vi "Elevator Controller.vi"(8 "error in":errorcluster) -> ()   [LabVIEW 2018]
doc: "This VI executes continuously carrying out the current operation and responding to updates or new operations. It will often contain the timing or control code that is difficult to place directly in TeleOp. This VI generally opens all sensors and motors and isolates the rest of the robot code from knowing how the operations are carried out."
uses:
  <vilib>/Rock Robotics/WPI/Framework/Completion Status.ctl
  Elevator Setpoints.ctl
  Elevator Operations.ctl
  <vilib>/Rock Robotics/WPI/ThirdParty/Phoenix-LabVIEW/Motor Controller/Controls/CTRE_Phoenix_MotorControl_FeedbackDevice.ctl
  <vilib>/Rock Robotics/WPI/ThirdParty/Phoenix-LabVIEW/Motor Controller/Controls/CTRE_Phoenix_MotorControl_LimitSwitchNormal.ctl
  <vilib>/Rock Robotics/WPI/ThirdParty/Phoenix-LabVIEW/Motor Controller/Controls/CTRE_Phoenix_MotorControl_LimitSwitchSource_Local.ctl
  <vilib>/Rock Robotics/WPI/ThirdParty/Phoenix-LabVIEW/Motor Controller/Controls/CTRE_Phoenix_MotorControl_ControlMode.ctl
  <vilib>/Rock Robotics/WPI/ThirdParty/Phoenix-LabVIEW/Motor Controller/Get/CTRE_Phoenix_MotorController_GetSelectedSensorData.vi
  <vilib>/Rock Robotics/Network Tables/NT Write Number.vi
  Elevator Published Globals.vi
  Framework/Robot Global Data.vi
  <vilib>/Rock Robotics/WPI/ThirdParty/Phoenix-LabVIEW/Motor Controller/Get/CTRE_Phoenix_MotorController_GetLimitSwitchStates.vi
  <vilib>/Rock Robotics/Network Tables/NT Write Boolean.vi
  <vilib>/Rock Robotics/WPI/ThirdParty/Phoenix-LabVIEW/Motor Controller/Get/CTRE_Phoenix_MotorController_GetClosedLoopData.vi
panel:
  in  "Time LimitDebounce":u32=500
  in  "ElevatorStopRange":dbl=20.0 format="%#_13g"
  out "Waveform Chart":i32(graph)
  out "inches":dbl=8.0
  out "% error":i32(graph)
  out "Position (Raw Sensor Units)":i32=208
  out "Waveform Chart 2":T1(graph)
  in  "Acceleration":i32=75
  in  "Cruise Velocity":i32=70
  in  "F":dbl=10.0
  in  "P":dbl=13.0
  in  "I":dbl
  in  "D":dbl
  in  "Interactive Values":T2={"Operation"=enum."LiftForTime", "Setpoint"=0.5, "Duration"=1.0, "Button"=FALSE}
  out "Current\nCmd":string="Started at  12:26:25.181\nDefault: Reserve,  S 0.0, D 0.000000"
  in  "Buttons":cluster{"Execute Cmd":bool, "Abort Cmd":bool}
  out "Command Timing":cluster{"Start Time (ms)":u32, "Iterations":i32}={"Start Time (ms)"=346916, "Iterations"=0}
  out "Status":T4=enum."Incomplete"
  # "Tip: It may be helpful to observe inputs and sensor values.\nYou may also want to display tuning or debugging controls."
  # "Interactive Command: You may fill in the settings for a command\nand schedule it with the Execute button. You can observe and abort\nany command while fine tuning the code for the controller."
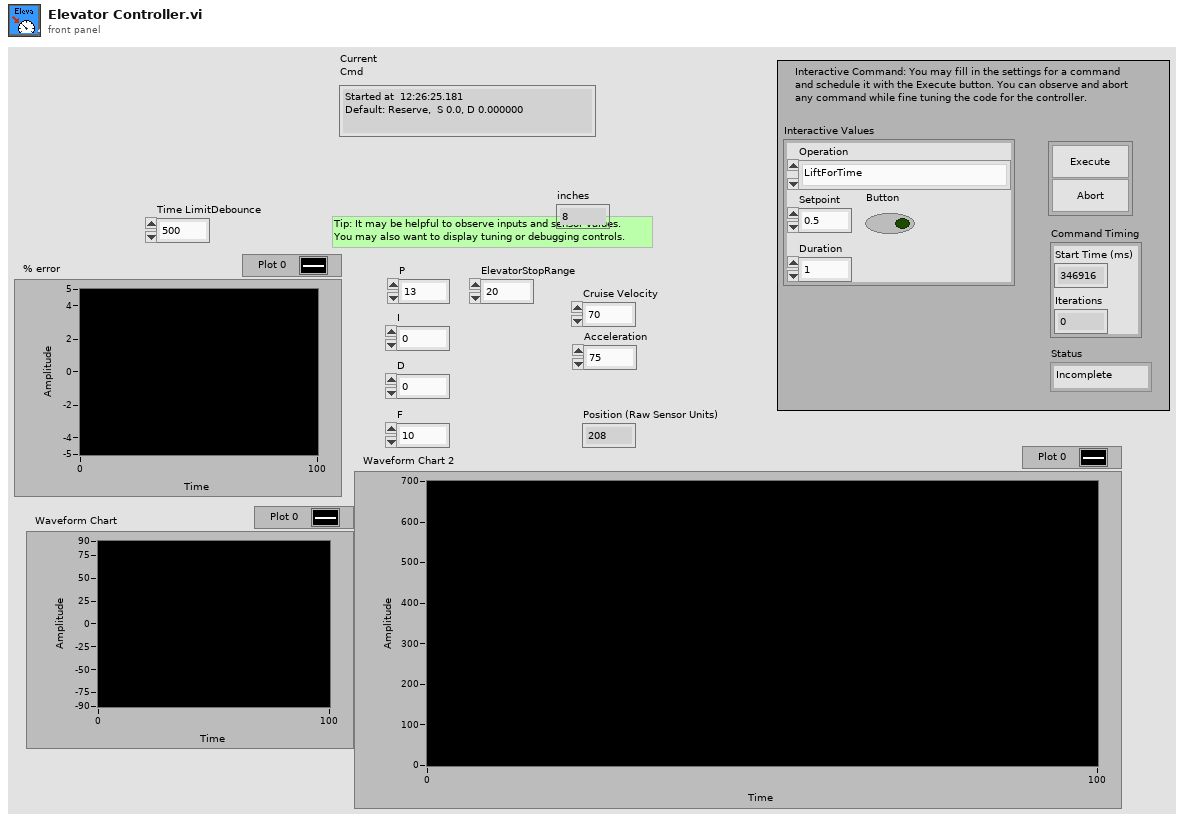
[diagram p1: front panel]
types:
  T1 = cluster{"Position (Raw Sensor Units)":i32, "Closed-loop Target":dbl}
  T2 = typedef "Elevator Setpoints.ctl" = cluster{"Operation":T3, "Setpoint":dbl, "Duration":dbl, "Button":bool}
  T3 = typedef "Elevator Operations.ctl" = enum16{"Reserve", "Read Current", "Immediate", "GoToHeight", "StayAtHeight", "LiftForTime"}
  T4 = typedef "Completion Status.ctl" = enum16{"Successful", "Aborted", "Incomplete"}
  T5 = typedef "CTRE_Phoenix_MotorControl_LimitSwitchSource_Local.ctl" = enum16{"Feedback Connector", "Remote Talon SRX", "Remote CANifier", "Deactivated"}
  T6 = typedef "CTRE_Phoenix_MotorControl_LimitSwitchNormal.ctl" = enum16{"Normally Open", "Normally Closed", "Disabled"}
  T7 = typedef "CTRE_Phoenix_MotorControl_FeedbackDevice.ctl" = i8
  T8 = typedef "WPI_MotorControlDeviceRef.ctl" = cluster{"DeviceStatus":errorcluster, "Type":T9, "PWM":cluster{"PWM Channel":T10, "DeadBand":T11}, "CAN":cluster{"Device Number":u8, "SetOutput VI Ref":variant, "GetOutput VI Ref":variant, "Enable VI Ref":variant, "Disable VI Ref":variant, "Data":variant}, "Invert":bool, "DIO PWM":cluster{"PWM \"Enable\" Channel":T10, "DIOChannel":T12, "PWM Rate":dbl}}
  T9 = typedef "WPI_MotorControlType.ctl" = enum16{"PWM", "CAN", "DIO PWM"}
  T10 = typedef "FPGA_DIOPWMChannel.ctl" = enum8{"PWM 0", "PWM 1", "PWM 2", "PWM 3", "PWM 4", "PWM 5", "PWM 6", "PWM 7", "PWM 8", "PWM 9", "PWM MXP 0", "PWM MXP 1", "PWM MXP 2", "PWM MXP 3", "PWM MXP 4", "PWM MXP 5", "PWM MXP 6", "PWM MXP 7", "PWM MXP 8", "PWM MXP 9", "Invalid"}
  T11 = typedef "WPI_PWMDeadband.ctl" = cluster{"Name":string, "maxPositivePwm":i32, "minPositivePwm":i32, "centerPwm":i32, "maxNegativePwm":i32, "minNegativePwm":i32, "angularRange":u16}
  T12 = typedef "FPGA_DIOChannel.ctl" = enum8{"DIO 0", "DIO 1", "DIO 2", "DIO 3", "DIO 4", "DIO 5", "DIO 6", "DIO 7", "DIO 8", "DIO 9", "DIO MXP 0", "DIO MXP 1", "DIO MXP 2", "DIO MXP 3", "DIO MXP 4", "DIO MXP 5", "DIO MXP 6", "DIO MXP 7", "DIO MXP 8", "DIO MXP 9", "DIO MXP 10", "DIO MXP 11", "DIO MXP 12", "DIO MXP 13", "DIO MXP 14", "DIO MXP 15", "SPI Port CS1", "SPI Port CS2", "SPI Port CS3", "SPI Port MISO", "SPI Port MOSI", "Invalid"}
  T13 = typedef "Command Status Info.ctl" = cluster{"Name":string, "Status":T4, "notifier out":T14}
  T14 = typedef "Completion Notifier.ctl" = refnum<notifier>
  T15 = cluster{"Current Command":T2, "Command Timing":cluster{"Start Time (ms)":u32, "Iterations":i32}, "Command Arguments":cluster{"Command Info":T13, "Description":string, "Default Command":T2, "queue out":refnum<queue>, "Subsystem Name":string}}
  T16 = typedef "CTRE_Phoenix_MotorControl_ControlMode.ctl" = u16
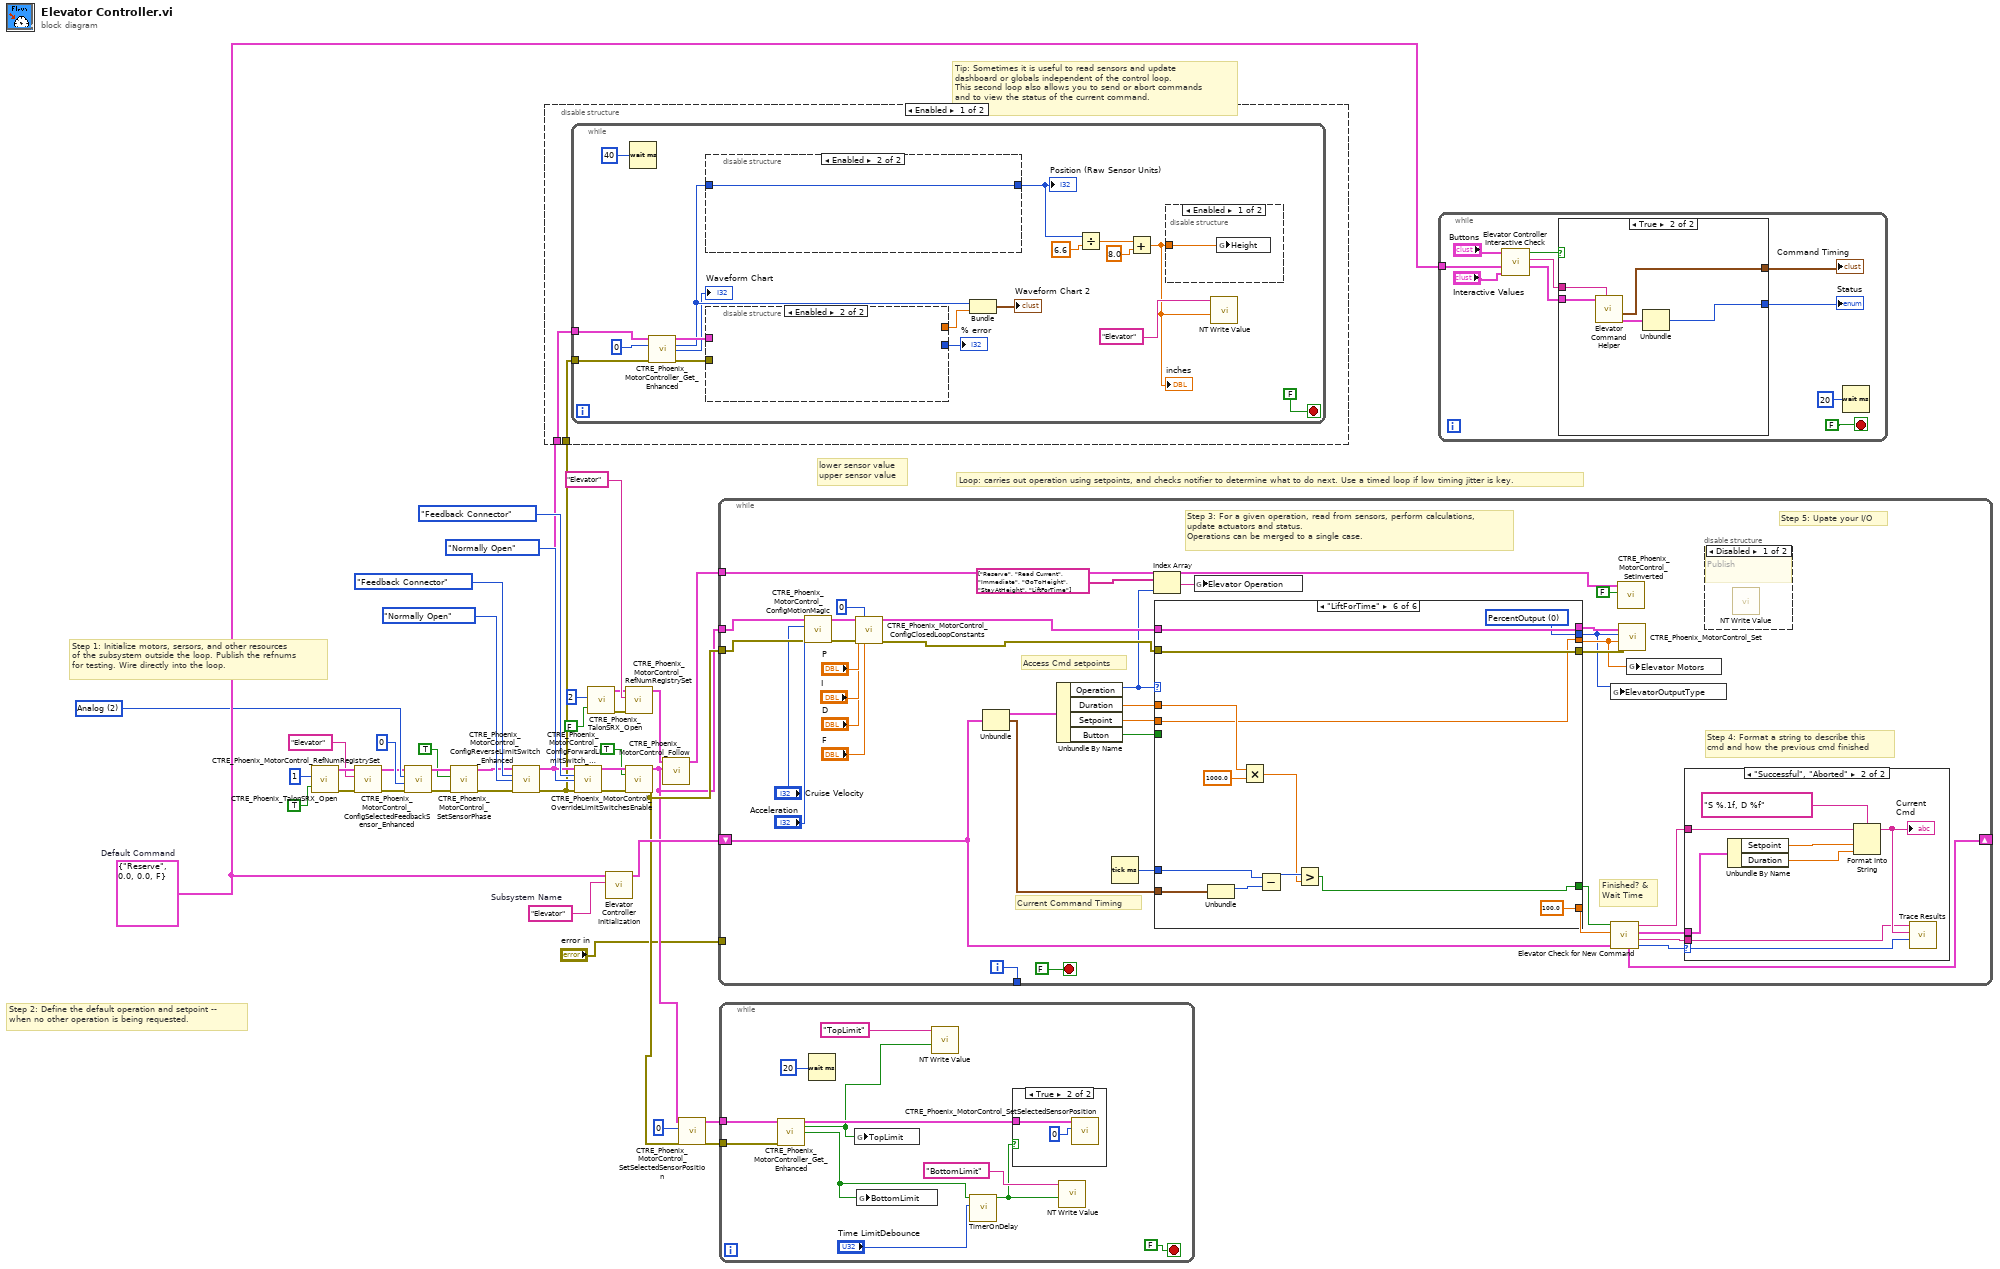
[diagram p0: block diagram]
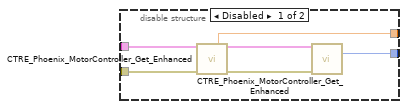
[diagram p3: hidden frame]
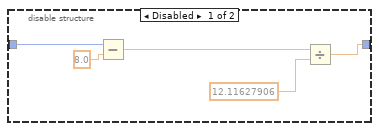
[diagram p5: hidden frame]
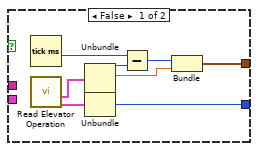
[diagram p7: hidden frame]
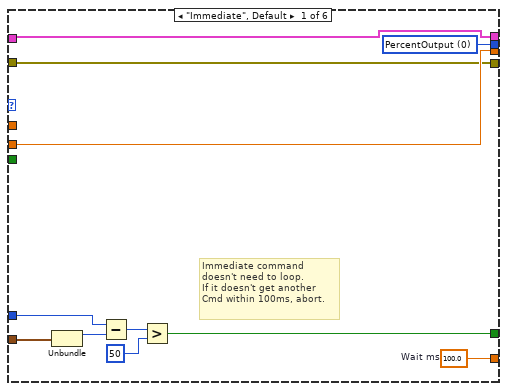
[diagram p10: hidden frame]
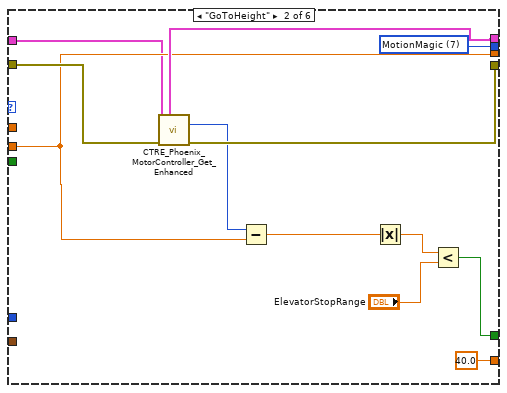
[diagram p11: hidden frame]
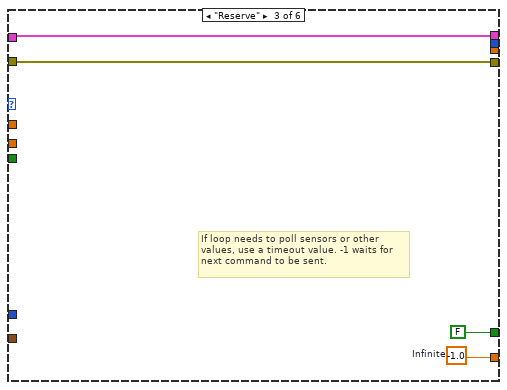
[diagram p12: hidden frame]
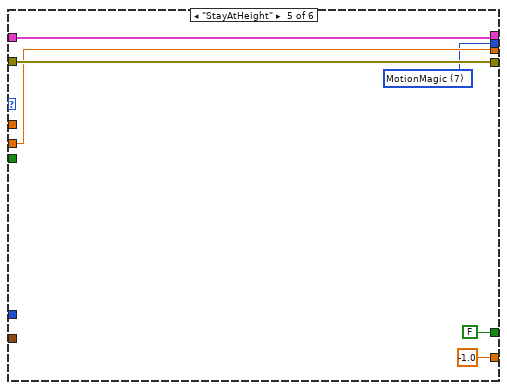
[diagram p14: hidden frame]
diagram:
  w30 = T7 2 items=["None"=-1, "QuadEncoder"=0, "Analog"=2, "Tachometer"=4, "Pulse Width Encoded Position"=8, "Sensor Sum (S0 + S1)"=9, "Sensor Difference (D0 - D1)"=10, "Remote Source 0"=11, "Remote Source 1"=12, "Software Emulated"=15] ("Feedback Device")
  w36 = T2 {"Operation"=enum."Reserve", "Setpoint"=0.0, "Duration"=0.0, "Button"=FALSE}  # Default Command
  w37 = "Elevator"  # Subsystem Name
  # "lower sensor value\nupper sensor value"
  # "Tip: Sometimes it is useful to read sensors and update\ndashboard or globals independent of the control loop.\nThis second loop also allows you to send or abort commands\nand to view the status of the current command."
  # "Step 2: Define the default operation and setpoint --\nwhen no other operation is being requested."
  # "Step 1: Initialize motors, sersors, and other resources\nof the subsystem outside the loop. Publish the refnums\nfor testing. Wire directly into the loop."
  # "Loop: carries out operation using setpoints, and checks notifier to determine what to do next. Use a timed loop if low timing jitter is key."
  n1 = call <vilib>:"CTRE_Phoenix_TalonSRX_Open.vi"("Invert"=TRUE, "Device Number"=u8 1) -> ("error out"=w34:errorcluster, "CAN Talon SRX Ref"=w35:T8)  [unwired: 8 in]
  n2 = call <vilib>:"CTRE_Phoenix_MotorControl_RefNumRegistrySet.vi"("error in (no error)"=w34, "refnum name"="Elevator", "PhoenixMotorControlDevRef"=w35) -> ("error out"=w31:errorcluster, "PhoenixMotorControlDevRef"=w13:T8)  [unwired: 7 in]
  n3 = call <vilib>:"CTRE_Phoenix_MotorControl_ConfigSelectedFeedbackSensor_Enhanced.vi"("error in (no error)"=w31, "pidLoopIdx"=0, "Feedback Device"=w30, "PhoenixMotorControlDevRef"=w13) -> ("error out"=w7:errorcluster, "PhoenixMotorControlDevRef"=w9:T8)  [unwired: 6 in]
  n4 = call <vilib>:"CTRE_Phoenix_MotorControl_SetSensorPhase.vi"("error in (no error)"=w7, "PhaseSensor"=TRUE, "PhoenixMotorControlDevRef"=w9) -> ("error out"=w6:errorcluster, "PhoenixMotorControlDevRef"=w8:T8)  [unwired: 7 in]
  n5 = call <vilib>:"CTRE_Phoenix_MotorControl_ConfigReverseLimitSwitch_Enhanced.vi"("PhoenixMotorControlDevRef"=w8, "Limit Switch Source"=CTRE_Phoenix_MotorControl_LimitSwitchSource_Local."Feedback Connector", "NormallyOpenOrClosed"=CTRE_Phoenix_MotorControl_LimitSwitchNormal."Normally Open", "error in (no error)"=w6) -> ("PhoenixMotorControlDevRef"=w21:T8, "error out"=w20:errorcluster)  [unwired: 10 in]
  n6 = disable-structure shown="Enabled" {
    disable-tunnel: w21 -> [w40 _]
    disable-tunnel: w20 -> [w39 _]
    frame Enabled {
      n7 = while {
        tunnel: w40 -> [w53]
        tunnel: w39 -> [w52]
        stop <- FALSE stop-if-true
        n8 = Wait (ms)(milliseconds to wait=u32 40) -> ()  [unwired: 1 out]
        n9 = call-poly <vilib>:"CTRE_Phoenix_MotorController_Get_Enhanced.vi"("PhoenixMotorControlDevRef"=w53, "pidLoopIdx"=u32 0, "error in"=w52) -> ("PhoenixMotorControlDevRef"=w57:T8, "Position (Raw Sensor Units)"=w48:i32, "Velocity (Raw Sensor Units per 100 ms)"=→"Waveform Chart":i32, "error out"=w51:errorcluster)  [unwired: 9 in]
        n10 = disable-structure shown="Enabled" {
          disable-tunnel: [w70 w71] -> w47
          disable-tunnel: w48 -> [w69 w71]
          frame Disabled {
            n11 = Subtract(x=w69, y=8.0) -> (x-y=w68:dbl)
            n12 = Divide(x=w68, y=12.11627906 ("x")) -> (x/y=w70:dbl)
          }
          frame Enabled {
          }
        }
        "Position (Raw Sensor Units)" <- w47
        n13 = disable-structure shown="Enabled" {
          disable-tunnel: w57 -> [w64 _]
          disable-tunnel: [w63 _] -> w56
          disable-tunnel: w51 -> [w62 _]
          disable-tunnel: [w59 _] -> w49
          frame Disabled {
            n14 = call-poly <vilib>:"CTRE_Phoenix_MotorController_Get_Enhanced.vi"("PhoenixMotorControlDevRef"=w64, "error in"=w62) -> ("Closed-loop Target"=w63:dbl, "PhoenixMotorControlDevRef"=w61:T8, "error out"=w60:errorcluster)  [unwired: 8 in, 3 out]
            n15 = call-poly <vilib>:"CTRE_Phoenix_MotorController_Get_Enhanced.vi"("PhoenixMotorControlDevRef"=w61, "error in"=w60) -> ("Closed-loop Error"=w59:i32)  [unwired: 8 in, 5 out]
          }
          frame Enabled {
          }
        }
        "% error" <- w49
        n16 = Bundle("Position (Raw Sensor Units)"=w48, "Closed-loop Target"=w56) -> (→"Waveform Chart 2":T1)  [unwired: 1 in]
        n17 = Divide(x=w47, y=6.6) -> (x/y=w44:dbl)
        n18 = Add(x=w44, y=8.0) -> (x+y=w41:dbl)
        "inches" <- w41
        n19 = disable-structure shown="Enabled" {
          disable-tunnel: w41 -> [w65 _]
          frame Enabled {
            n20 = global write "Elevator Published Globals.vi" "Height"(w65) -> ()
          }
          frame Disabled {
          }
        }
        n21 = call-poly <vilib>:"NT Write Value.vi"("Numeric"=w41, "Name"="Elevator") -> ()  [unwired: 9 in, 1 out]
      }
    }
    frame Disabled {
    }
  }
  n22 = call <vilib>:"CTRE_Phoenix_MotorControl_ConfigForwardLimitSwitch_Enhanced.vi"("PhoenixMotorControlDevRef"=w21, "Limit Switch Source"=CTRE_Phoenix_MotorControl_LimitSwitchSource_Local."Feedback Connector", "NormallyOpenOrClosed"=CTRE_Phoenix_MotorControl_LimitSwitchNormal."Normally Open", "error in (no error)"=w20) -> ("PhoenixMotorControlDevRef"=w24:T8, "error out"=w23:errorcluster)  [unwired: 10 in]
  n23 = call <vilib>:"CTRE_Phoenix_TalonSRX_Open.vi"("Invert"=FALSE, "Device Number"=u8 2) -> ("error out"=w17:errorcluster, "CAN Talon SRX Ref"=w16:T8)  [unwired: 8 in]
  n24 = call "Elevator Controller Initialization.vi"("Subsystem Name"=w37, "Default Command"=w36) -> ("Current Command"=w38:T15)  [unwired: 9 in]
  n25 = call <vilib>:"CTRE_Phoenix_MotorControl_RefNumRegistrySet.vi"("error in (no error)"=w17, "refnum name"="Elevator", "PhoenixMotorControlDevRef"=w16) -> ("PhoenixMotorControlDevRef"=w12:T8)  [unwired: 7 in, 1 out]
  n26 = call <vilib>:"CTRE_Phoenix_MotorControl_OverrideLimitSwitchesEnable.vi"("PhoenixMotorControlDevRef"=w24, "Override Limit Switch Enable?"=TRUE, "error in (no error)"=w23) -> ("PhoenixMotorControlDevRef"=w3:T8, "error out"=w10:errorcluster)  [unwired: 11 in]
  n27 = call <vilib>:"CTRE_Phoenix_MotorControl_Follow.vi"("Master Controller to Follow"=w3, "PhoenixMotorControlDevRef"=w12) -> ("PhoenixMotorControlDevRef"=w11:T8)  [unwired: 8 in, 1 out]
  n28 = call <vilib>:"CTRE_Phoenix_MotorControl_SetSelectedSensorPosition.vi"("New Sensor Position"=0, "PhoenixMotorControlDevRef"=w3) -> ("PhoenixMotorControlDevRef"=w2:T8)  [unwired: 8 in, 1 out]
  n29 = while {
    shift-right: [w103] -> _
    shift-left: w38 -> [w96]
    tunnel: [w108] -> _
    tunnel: "error in" -> [_]
    tunnel: w3 -> [w79]
    tunnel: w10 -> [w84]
    tunnel: w11 -> [w77]
    i -> [w108]
    stop <- FALSE stop-if-true
    # "Step 5: Upate your I/O"
    # "Step 4: Format a string to describe this\ncmd and how the previous cmd finished"
    # "Current Command Timing"
    # "Access Cmd setpoints"
    # "Finished? &\nWait Time"
    # "Step 3: For a given operation, read from sensors, perform calculations,\nupdate actuators and status.\nOperations can be merged to a single case."
    n30 = call <vilib>:"CTRE_Phoenix_MotorControl_ConfigMotionMagic.vi"("error in (no error)"=w84, "Acceleration"="Acceleration", "Cruise Velocity"="Cruise Velocity", "PhoenixMotorControlDevRef"=w79) -> ("error out"=w89:errorcluster, "PhoenixMotorControlDevRef"=w88:T8)  [unwired: 6 in]
    n31 = call <vilib>:"CTRE_Phoenix_MotorControl_ConfigClosedLoopConstants.vi"("PhoenixMotorControlDevRef"=w88, "slotIdx"=0, "P"="P", "I"="I", "D"="D", "error in (no error)"=w89, "F"="F") -> ("PhoenixMotorControlDevRef"=w81:T8, "error out"=w80:errorcluster)  [unwired: 7 in]
    n32 = Unbundle(w96) -> ("Current Command"=w107:T2, "Command Timing"=w105:cluster{"Start Time (ms)":u32, "Iterations":i32})  [unwired: 1 out]
    n33 = Unbundle By Name(w107) -> ("Operation"=w74:T3, "Duration"=w106:dbl, "Setpoint"=w104:dbl, "Button"=w83:bool)
    n34 = Tick Count (ms)() -> (millisecond timer value=w95:u32)
    n35 = Index Array(array=string[] ["Reserve", "Read Current", "Immediate", "GoToHeight", "StayAtHeight", "LiftForTime"] ("Strings []"), index=w74) -> (element=w73:string)
    n36 = case shown="\"LiftForTime\"" w74 {
      tunnel: [w128 40.0 ("Infinite") w144 _ -1.0 ("Infinite") 100.0 ("Infinite")] -> w101
      tunnel: [w122 w129 FALSE ("ignore previous (F)") _ FALSE ("ignore previous (F)") w158] -> w102
      tunnel: w105 -> [w124 _ _ _ _ w159]
      tunnel: w106 -> [_ _ _ _ _ w156]
      tunnel: w104 -> [w120 w131 _ _ w150 w153]
      tunnel: w81 -> [w118 w130 w142 w146 w152 w165]
      tunnel: w80 -> [w119 w138 w141 w145 w151 w164]
      tunnel: w95 -> [w123 _ _ _ _ w160]
      tunnel: [w119 w136 w141 w145 w151 w164] -> w94
      tunnel: [w118 w137 w142 w146 w152 w165] -> w93
      tunnel: [w120 w131 _ _ w150 w153] -> w76
      tunnel: [w121 w140 _ _ w148 w163] -> w75
      tunnel: w83 -> [_ _ _ _ _ _]
      frame "Immediate", Default {
        w121 = T16 0 items=["PercentOutput"=0, "Position"=1, "Velocity"=2, "Current"=3, "Follower"=5, "MotionProfile"=6, "MotionMagic"=7, "MotionMagicArc"=8, "MotionProfileArc"=10, "Disabled"=15] ("Control Mode")
        w128 = 100.0  # Wait ms
        # "Immediate command\ndoesn't need to loop.\nIf it doesn't get another\nCmd within 100ms, abort."
        n37 = Unbundle(w124) -> ("Start Time (ms)"=w127:u32)  [unwired: 1 out]
        n38 = Subtract(x=w123, y=w127) -> (x-y=w126:u32)
        n39 = Greater?(x=w126, y=u8 50 ("Left Motor")) -> (0:w122:bool)
      }
      frame "GoToHeight" {
        w140 = T16 7 items=["PercentOutput"=0, "Position"=1, "Velocity"=2, "Current"=3, "Follower"=5, "MotionProfile"=6, "MotionMagic"=7, "MotionMagicArc"=8, "MotionProfileArc"=10, "Disabled"=15] ("Control Mode")
        n40 = call-poly <vilib>:"CTRE_Phoenix_MotorController_Get_Enhanced.vi"("PhoenixMotorControlDevRef"=w130, "error in"=w138) -> ("PhoenixMotorControlDevRef"=w137:T8, "Position (Raw Sensor Units)"=w132:i32, "error out"=w136:errorcluster)  [unwired: 10 in, 1 out]
        n41 = Subtract(x=w132, y=w131) -> (x-y=w135:dbl)
        n42 = Absolute Value(x=w135) -> (abs(x)=w134:dbl)
        n43 = Less?(x=w134, y="ElevatorStopRange") -> (x < y?=w129:bool)
      }
      frame "Reserve" {
        w144 = -1.0  # Infinite
        # "If loop needs to poll sensors or other\nvalues, use a timeout value. -1 waits for\nnext command to be sent."
      }
      frame "Read Current" {
      }
      frame "StayAtHeight" {
        w148 = T16 7 items=["PercentOutput"=0, "Position"=1, "Velocity"=2, "Current"=3, "Follower"=5, "MotionProfile"=6, "MotionMagic"=7, "MotionMagicArc"=8, "MotionProfileArc"=10, "Disabled"=15] ("Control Mode")
      }
      frame "LiftForTime" {
        w163 = T16 0 items=["PercentOutput"=0, "Position"=1, "Velocity"=2, "Current"=3, "Follower"=5, "MotionProfile"=6, "MotionMagic"=7, "MotionMagicArc"=8, "MotionProfileArc"=10, "Disabled"=15] ("Control Mode")
        n44 = Unbundle(w159) -> ("Start Time (ms)"=w161:u32)  [unwired: 1 out]
        n45 = Multiply(x=w156, y=1000.0) -> (x*y=w155:dbl)
        n46 = Subtract(x=w160, y=w161) -> (x-y=w162:u32)
        n47 = Greater?(x=w162, y=w155) -> (0:w158:bool)
      }
    }
    n48 = global write "Robot Global Data.vi" "Elevator Operation"(w73) -> ()
    n49 = global write "Robot Global Data.vi" "ElevatorOutputType"(w75) -> ()
    n50 = call "Elevator Check for New Command.vi"("Current Command"=w96, "Wait time (ms)"=w101, "Finished?"=w102) -> ("Completion"=w97:T4, "Subsystem Name"=w98:string, "Current Command"=w99:T2, "Initial Trace String"=w100:string, "NextCommand"=w103:T15)  [unwired: 4 in]
    n51 = call <vilib>:"CTRE_Phoenix_MotorControl_SetInverted.vi"("Invert?"=FALSE, "PhoenixMotorControlDevRef"=w77) -> ()  [unwired: 8 in, 2 out]
    n52 = call <vilib>:"CTRE_Phoenix_MotorControl_Set.vi"("error in (no error)"=w94, "Output"=w76, "Control Mode"=w75, "PhoenixMotorControlDevRef"=w93) -> ()  [unwired: 6 in, 2 out]
    n53 = global write "Robot Global Data.vi" "Elevator Motors"(w76) -> ()
    n54 = case shown="\"Successful\", \"Aborted\"" w97 {
      selector: w97 -> [_ w117]
      tunnel: w100 -> [_ w113]
      tunnel: w99 -> [_ w114]
      tunnel: w98 -> [_ w110]
      frame "Incomplete", Default {
        # "Continuing current command"
      }
      frame "Successful", "Aborted" {
        # "Report and setup for next command"
        n55 = Unbundle By Name(w114) -> ("Setpoint"=w116:dbl, "Duration"=w111:dbl)
        n56 = Format Into String(format string="S %.1f, D %f", initial string=w113, w116, w111) -> (resulting string=w112:string)  [unwired: 1 in, 1 out]
        "Current\nCmd" <- w112
        n57 = call <vilib>:"Trace Results.vi"("Status of previous command"=w117, "Description"=w112, "Subsystem"=w110) -> ()  [unwired: 9 in]
      }
    }
    n58 = disable-structure shown="Disabled" {
      frame Disabled {
        # "Publish"
        n59 = call-poly <vilib>:"NT Write Value.vi"() -> ()  [unwired: 11 in, 1 out]
      }
      frame Enabled {
      }
    }
  }
  n60 = while {
    tunnel: w2 -> [w175]
    tunnel: w10 -> [w176]
    stop <- FALSE stop-if-true
    n61 = call-poly <vilib>:"CTRE_Phoenix_MotorController_Get_Enhanced.vi"("PhoenixMotorControlDevRef"=w175, "error in"=w176) -> ("PhoenixMotorControlDevRef"=w173:T8, "Forward Limit Closed?"=w166:bool, "Reverse Limit Closed?"=w167:bool)  [unwired: 10 in, 1 out]
    n62 = Wait (ms)(milliseconds to wait=u32 20 ("millisecond timer value")) -> ()  [unwired: 1 out]
    n63 = global write "Elevator Published Globals.vi" "TopLimit"(w166) -> ()
    n64 = global write "Elevator Published Globals.vi" "BottomLimit"(w167) -> ()
    n65 = call-poly <vilib>:"NT Write Value.vi"("Boolean"=w166, "Name"="TopLimit") -> ()  [unwired: 9 in, 1 out]
    n66 = call "TimerOnDelay.vi"("Time Limit"="Time LimitDebounce", "Input"=w167) -> ("Output"=w169:bool)  [unwired: 9 in]
    n67 = case shown="True" w169 {
      tunnel: w173 -> [_ w178]
      frame False {
      }
      frame True {
        n68 = call <vilib>:"CTRE_Phoenix_MotorControl_SetSelectedSensorPosition.vi"("New Sensor Position"=0, "PhoenixMotorControlDevRef"=w178) -> ()  [unwired: 8 in, 2 out]
      }
    }
    n69 = call-poly <vilib>:"NT Write Value.vi"("Boolean"=w169, "Name"="BottomLimit") -> ()  [unwired: 9 in, 1 out]
  }
  n70 = while {
    tunnel: w36 -> [w185]
    stop <- FALSE stop-if-true
    n71 = call "Elevator Controller Interactive Check.vi"("Interactive Command in"="Interactive Values", "Default Command"=w185, "Buttons"="Buttons") -> ("Interactive Command out"=w182:T2, "Trace String"=w183:string, "Schedule"=w184:bool)  [unwired: 6 in]
    n72 = case shown="True" w184 {
      tunnel: [w196 w201] -> w181
      tunnel: w182 -> [_ w199]
      tunnel: [w192 w197] -> w180
      tunnel: w183 -> [_ w200]
      frame False {
        n73 = Tick Count (ms)() -> (millisecond timer value=w191:u32)
        n74 = call "Read Elevator Operation.vi"() -> ("Command Info"=w189:T13, "SubSystem Data"=w190:T2)  [unwired: 9 in, 1 out]
        n75 = Unbundle(w190) -> ("Operation"=w195:T3, "Setpoint"=w193:dbl)  [unwired: 2 out]
        n76 = Unbundle(w189) -> ("Status"=w196:T4)  [unwired: 2 out]
        n77 = Subtract(x=w191, y=w195) -> (x-y=w194:u32)
        n78 = Bundle(w194, "Setpoint"=w193) -> (w192:cluster{u32, "Setpoint":dbl})  [unwired: 1 in]
      }
      frame True {
        n79 = call "Elevator Command Helper.vi"("Description"=w200, "SubSystem Data"=w199) -> ("Command Info Out"=w198:T13, "Command Timing"=w197:cluster{"Start Time (ms)":u32, "Iterations":i32})  [unwired: 7 in, 1 out]
        n80 = Unbundle(w198) -> ("Status"=w201:T4)  [unwired: 2 out]
      }
    }
    "Status" <- w181
    "Command Timing" <- w180
    n81 = Wait (ms)(milliseconds to wait=u32 20) -> ()  [unwired: 1 out]
  }
